vi "Close HIL Mode.vi"(8 "error in":errorcluster) -> (0 "error out":errorcluster)   [LabVIEW 2017, in "DTACQ - Network Enabled Device Driver.lvlib"]
doc: "Closes the connections to the shared variables"
uses:
  DTACQ - Network Enabled Device Driver.lvlib
  FGV Operaions--Enum.ctl
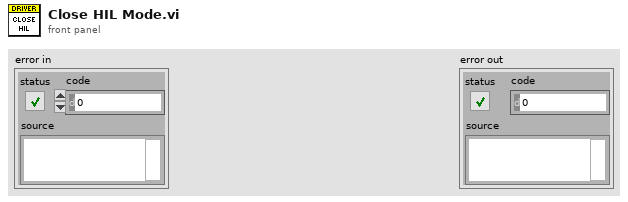
[diagram p1: front panel]
types:
  T1 = typedef "DTACQ - Network Enabled Device Driver.lvlib/FGV Operaions--Enum.ctl" = enum16{"Get Driver Settings", "Set Driver Settings", "Search Variable Names", "Close Connections", "Open Connections", "Get Variable References", "Set Variable References", "Clear"}
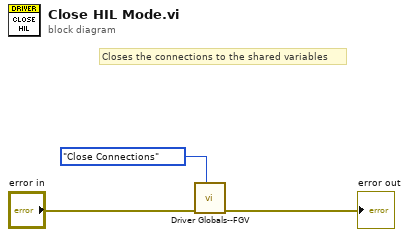
[diagram p0: block diagram]
diagram:
  # "Closes the connections to the shared variables"
  n1 = call "Driver Globals--FGV.vi"(7:FGV_Operaions--Enum."Close Connections", "error in"="error in") -> ("error out"=→"error out":errorcluster)  [unwired: 6 in, 3 out]
